vi "Read Sequencer State.vi"(8 "error in (no error)":errorcluster, 11 "Simple Sequencer in":refnum<class "Simple Sequencer.lvclass">) -> (0 "error out":errorcluster, 2 "Sequencer state":T1, 3 "Simple Sequencer out":refnum<class "Simple Sequencer.lvclass">)   [LabVIEW 2018, in "Simple Sequencer.lvclass"]
uses:
  Simple Sequencer.lvclass
  NHMFL_Core/Libraries/Instruments/Sequence/Sequencer State Machine/Sequencer State.ctl
  Simple Sequencer.lvclass/Simple Sequencer.ctl
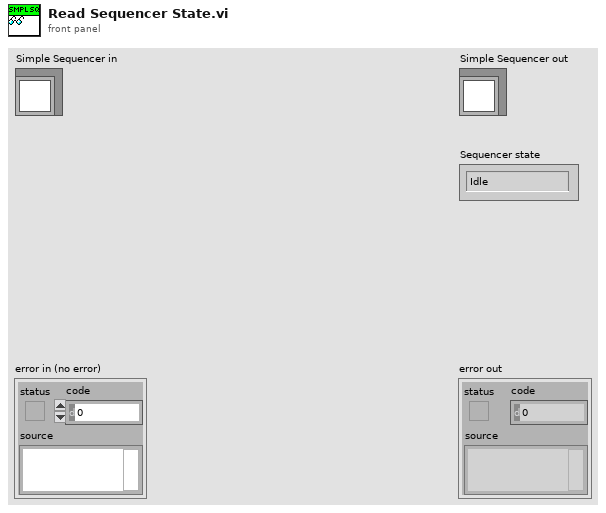
[diagram p1: front panel]
types:
  T1 = typedef "Sequencer State.ctl" = enum16{"Idle", "Starting", "Waiting for primary", "Waiting for secondary"}
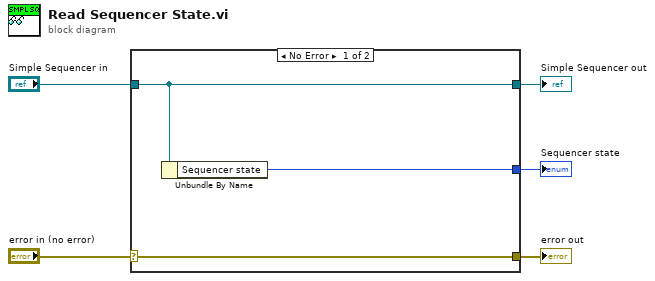
[diagram p0: block diagram]
diagram:
  n1 = case shown="No Error" "error in (no error)" {
    selector: "error in (no error)" -> [w8 w9]
    tunnel: [w8 w9] -> w4
    tunnel: [w7 w10] -> w2
    tunnel: "Simple Sequencer in" -> [w7 w10]
    tunnel: [w6 _] -> w1
    frame No Error {
      n2 = Unbundle By Name(w7) -> ("Sequencer state"=w6:T1)
    }
    frame Error {
    }
  }
  "error out" <- w4
  "Simple Sequencer out" <- w2
  "Sequencer state" <- w1
